vi "AlazarGetParameter.vi"(4 "error in (no error)":errorcluster, 5 "Parameter":u32(ring)=268435465 items=["Data Width"=268435465, "Set/Get Async BuffSize"=268435513, "Set/Get Async Buffcount"=268435520, "Get Data Format"=268435522, "Get Samples Per Timestamp Clock"=268435524, "Get Records Captured"=268435525, "Get Async Buffers Pending"=268435536, "Get Async Buffers Pending Full"=268435537, "Get Async Buffers Pending Empty"=268435538, "ECC Mode"=268435528, "Get Aux Input Level"=268435529, "Get Channels Per Board"=268435568, "Pack Mode"=268435570, "Get FPGA Temperature"=268435584], 6 "Channel":u8(ring)=1 items=["A"=1, "B"=2, "C"=4, "D"=8], 7 "Handle":u32) -> (0 "error out":errorcluster, 1 "Return Code":u32, 2 "Value":i32, 3 "Handle":u32)   [LabVIEW 2021]
doc: "Get a device attribute as a signed long value."
uses:
  ATSApi.dll
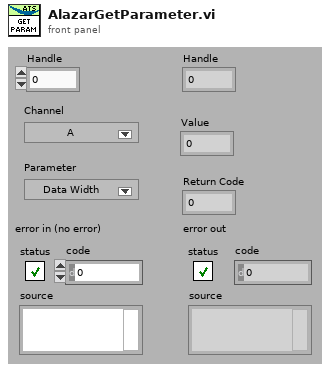
[diagram p1: front panel]
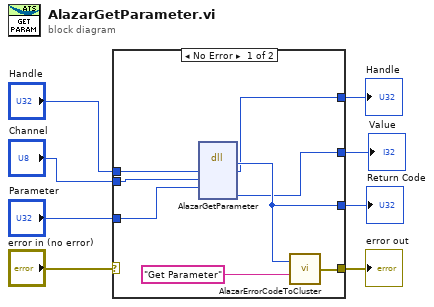
[diagram p0: block diagram]
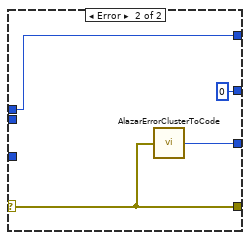
[diagram p2: hidden frame]
diagram:
  n1 = case shown="No Error" "error in (no error)" {
    selector: "error in (no error)" -> [_ w20]
    tunnel: [w13 w20] -> w7
    tunnel: [w15 w19] -> w6
    tunnel: "Handle" -> [w16 w18]
    tunnel: [w12 w18] -> w4
    tunnel: "Channel" -> [w11 _]
    tunnel: "Parameter" -> [w10 _]
    tunnel: [w9 0] -> w1
    frame No Error {
      n2 = dll-call lib="ATSApi.dll" fn="AlazarGetParameter"("handle"=w16, "Channel"=w11, "Parameter"=w10) -> (w15:u32, "handle"=w12:u32, "Value"=w9:i32)  [unwired: 6 in, 2 out]
      n3 = call "AlazarErrorCodeToCluster.vi"("Message"="Get Parameter", "Error Code"=w15) -> ("error out"=w13:errorcluster)
    }
    frame Error {
      n4 = call "AlazarErrorClusterToCode.vi"("error in (no error)"=w20) -> ("Error Code"=w19:u32)
    }
  }
  "Handle" <- w4
  "error out" <- w7
  "Return Code" <- w6
  "Value" <- w1
